vi "konfig lesen.vi"() -> ()   [LabVIEW 2010]
panel:
  out "Werte1":i32[](array[numeric])
  out "Werte2":dbl[](array[numeric])
  out "Werte3":i32[](array[numeric])
  out "Parameter3":string
  out "Parameter2":string
  out "Parameter1":string
  in  "Konfigurationsdatei auswählen":path
  out "Konfiguration":string
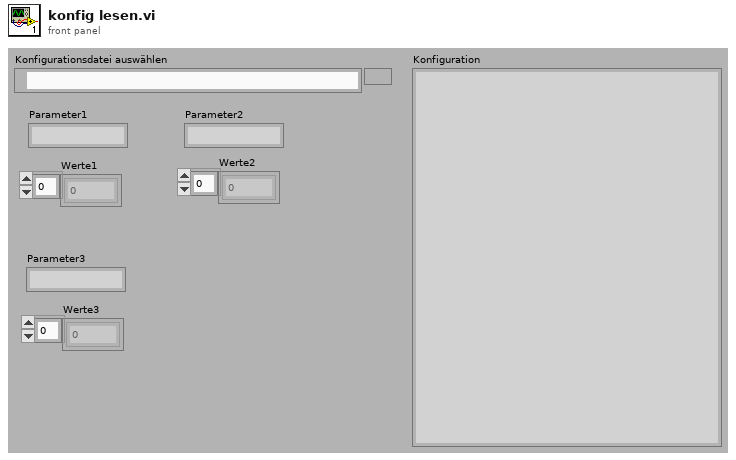
[diagram p1: front panel]
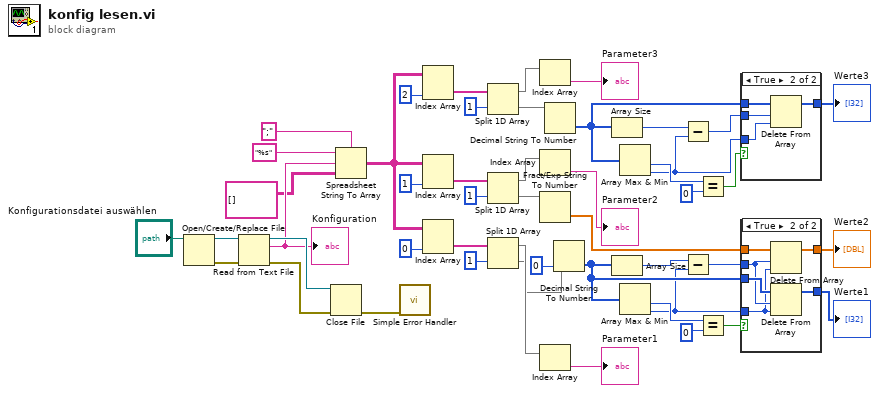
[diagram p0: block diagram]
diagram:
  n1 = Open/Create/Replace File(file path (use dialog)="Konfigurationsdatei auswählen") -> (refnum out=w48:refnum<file>, error out=w47:errorcluster)  [unwired: 5 in, 1 out]
  n2 = Read from Text File(file (use dialog)=w48, error in=w47) -> (refnum out=w45:refnum<file>, text=w42:string, error out=w46:errorcluster)  [unwired: 2 in, 1 out]
  "Konfiguration" <- w42
  n3 = Close File(refnum=w45, error in=w46) -> (error out=w44:errorcluster)  [unwired: 1 out]
  n4 = Spreadsheet String To Array(delimiter (Tab)=";" ("Trennzeichen (Tabulator)"), format string="%s" ("Format-String"), spreadsheet string=w42, array type (2D Dbl)=string[][] []) -> (array=w6:string[][])
  n5 = call <vilib>:"Simple Error Handler.vi"("error in (no error)"=w44) -> ()  [unwired: 4 in, 5 out]
  n6 = Index Array(array=w6, index (col)=2 ("Index")) -> (element=w23:string[])  [unwired: 1 in]
  n7 = Index Array(array=w6, index (col)=1 ("Index")) -> (element=w14:string[])  [unwired: 1 in]
  n8 = Index Array(array=w6, index (col)=0 ("Index")) -> (element=w8:string[])  [unwired: 1 in]
  n9 = Split 1D Array(array=w23, index=1 ("Index")) -> (first subarray=w20:string[], second subarray=w21:string[])
  n10 = Split 1D Array(array=w14, index=1 ("Index")) -> (first subarray=w12:string[], second subarray=w10:string[])
  n11 = Split 1D Array(array=w8, index=1 ("Index")) -> (first subarray=w2:string[], second subarray=w1:string[])
  n12 = Index Array(array=w20) -> (element=→"Parameter3":string)  [unwired: 1 in]
  n13 = Index Array(array=w12) -> (element=→"Parameter2":string)  [unwired: 1 in]
  n14 = Fract/Exp String To Number(string=w10) -> (number=w27:dbl[])  [unwired: 3 in, 1 out]
  n15 = Index Array(array=w2) -> (element=→"Parameter1":string)  [unwired: 1 in]
  n16 = Decimal String To Number(string=w21) -> (number=w25:i32[])  [unwired: 2 in, 1 out]
  n17 = Decimal String To Number(string=w1, default (0L)=0 ("Standard (0 I32)")) -> (number=w29:i32[])  [unwired: 1 in, 1 out]
  n18 = Array Size(array=w25) -> (size(s)=w18:i32)
  n19 = Array Size(array=w29) -> (size(s)=w4:i32)
  n20 = Array Max & Min(array=w25) -> (min value=w37:i32, min index (indices)=w17:i32)  [unwired: 2 out]
  n21 = Array Max & Min(array=w29) -> (min value=w33:i32, min index (indices)=w3:i32)  [unwired: 2 out]
  n22 = Subtract(x=w18, y=w17) -> (x-y=w34:i32)
  n23 = Subtract(x=w4, y=w3) -> (x-y=w30:i32)
  n24 = Equal?(x=w37, y=0) -> (x = y?=w35:bool)
  n25 = Equal?(x=w33, y=0) -> (x = y?=w31:bool)
  n26 = case shown="True" w35 {
    tunnel: w25 -> [w49 w53]
    tunnel: w17 -> [_ w51]
    tunnel: [w49 w52] -> w16
    tunnel: w34 -> [_ w50]
    frame False {
    }
    frame True {
      n27 = Delete From Array(array=w53, length=w50, index=w51) -> (array with subset deleted=w52:i32[])  [unwired: 1 out]
    }
  }
  "Werte3" <- w16
  n28 = case shown="True" w31 {
    tunnel: w29 -> [w55 w61]
    tunnel: w3 -> [_ w56]
    tunnel: [w55 w60] -> w28
    tunnel: w30 -> [_ w57]
    tunnel: w27 -> [w54 w59]
    tunnel: [w54 w58] -> w26
    frame False {
    }
    frame True {
      n29 = Delete From Array(array=w59, length=w57, index=w56) -> (array with subset deleted=w58:dbl[])  [unwired: 1 out]
      n30 = Delete From Array(array=w61, length=w57, index=w56) -> (array with subset deleted=w60:i32[])  [unwired: 1 out]
    }
  }
  "Werte2" <- w26
  "Werte1" <- w28
